vi "Make URL.vi"(7 "Port":T1(ring), 10 "Connection Info":T2) -> (2 "Connection URL":string)   [LabVIEW 2018, in "ClientMessaging.lvlib"]
uses:
  ClientMessaging.lvlib
  Connection.ctl
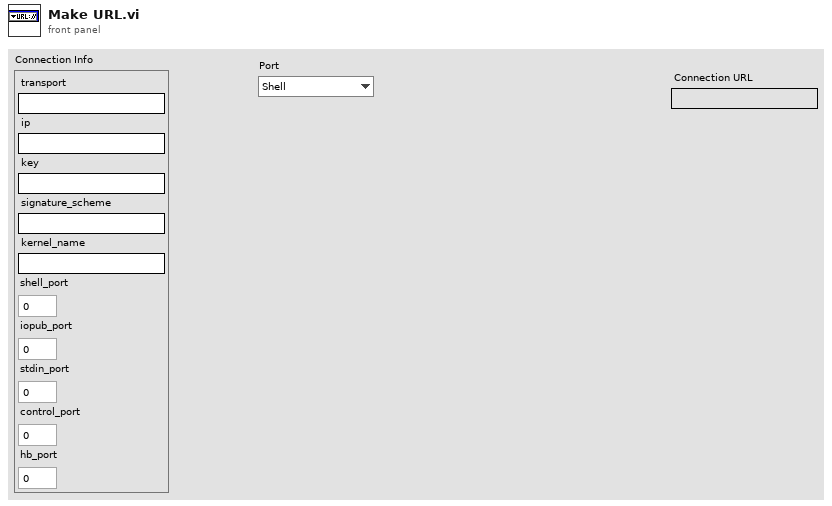
[diagram p1: front panel]
types:
  T1 = enum16{"Shell", "IOPub", "Stdin", "Control", "Heart Beat"}
  T2 = typedef "ClientMessaging.lvlib/Connection.ctl" = cluster{"transport":string, "ip":string, "key":string, "signature_scheme":string, "kernel_name":string, "shell_port":u16, "iopub_port":u16, "stdin_port":u16, "control_port":u16, "hb_port":u16}
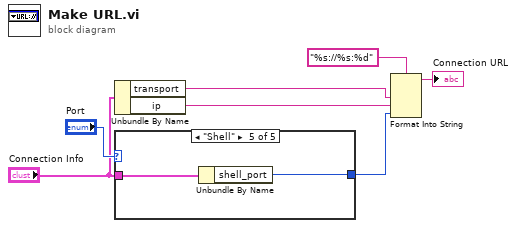
[diagram p0: block diagram]
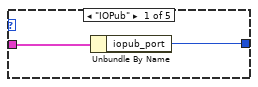
[diagram p2: hidden frame]
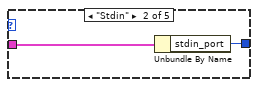
[diagram p3: hidden frame]
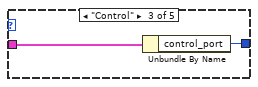
[diagram p4: hidden frame]
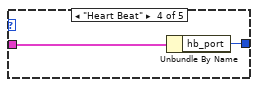
[diagram p5: hidden frame]
diagram:
  n1 = Unbundle By Name("Connection Info") -> ("transport"=w5:string, "ip"=w4:string)
  n2 = case shown="\"Shell\"" "Port" {
    tunnel: [w9 w11 w13 w15 w17] -> w3
    tunnel: "Connection Info" -> [w8 w10 w12 w14 w16]
    frame "IOPub" {
      n3 = Unbundle By Name(w8) -> ("iopub_port"=w9:u16)
    }
    frame "Stdin" {
      n4 = Unbundle By Name(w10) -> ("stdin_port"=w11:u16)
    }
    frame "Control" {
      n5 = Unbundle By Name(w12) -> ("control_port"=w13:u16)
    }
    frame "Heart Beat" {
      n6 = Unbundle By Name(w14) -> ("hb_port"=w15:u16)
    }
    frame "Shell" {
      n7 = Unbundle By Name(w16) -> ("shell_port"=w17:u16)
    }
  }
  n8 = Format Into String(format string="%s://%s:%d", w5, w4, w3) -> (resulting string=→"Connection URL":string)  [unwired: 2 in, 1 out]
